vi "DateToHex.vi"(11 "DATE":timestamp[](array[timestamp])) -> (3 "数组":u16[](array[numeric]) format="%04xH")   [LabVIEW 2016, in "斯坦道总磷总氮V2.lvlib"]
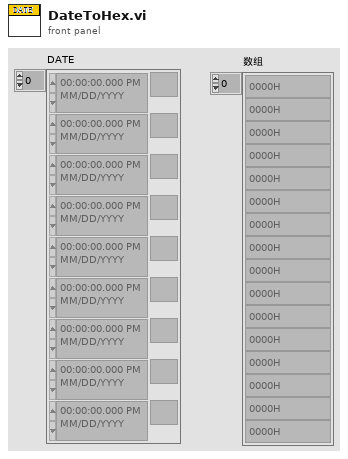
[diagram p1: front panel]
types:
  T1 = typedef "LVDateTimeRec.ctl" = cluster{"秒数的小数部分":dbl, "秒":i32, "分":i32, "时":i32, "日":i32, "月":i32, "年":i32, "天数（周）":i32, "天数（年）":i32, "DST":i32}
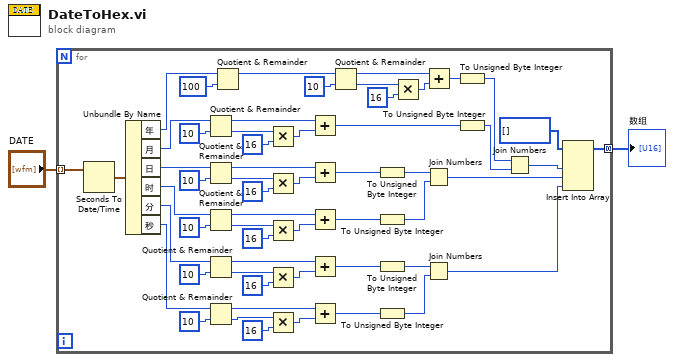
[diagram p0: block diagram]
diagram:
  n1 = for {
    tunnel: "DATE" -> [w59] mode=indexing
    tunnel: [w3] -> w1 mode=concatenating
    n2 = Seconds To Date/Time(time stamp (now)=w59) -> (date time rec=w58:T1)  [unwired: 1 in]
    n3 = Unbundle By Name(w58) -> ("年"=w26:i32, "月"=w14:i32, "日"=w13:i32, "时"=w12:i32, "分"=w11:i32, "秒"=w10:i32)
    n4 = Quotient & Remainder(x=w14, y=10) -> (x-y*floor(x/y)=w33:i32, floor(x/y)=w36:i32)
    n5 = Quotient & Remainder(x=w13, y=10) -> (x-y*floor(x/y)=w43:i32, floor(x/y)=w46:i32)
    n6 = Quotient & Remainder(x=w12, y=10) -> (x-y*floor(x/y)=w42:i32, floor(x/y)=w39:i32)
    n7 = Quotient & Remainder(x=w11, y=10) -> (x-y*floor(x/y)=w53:i32, floor(x/y)=w56:i32)
    n8 = Quotient & Remainder(x=w10, y=10) -> (x-y*floor(x/y)=w52:i32, floor(x/y)=w49:i32)
    n9 = Quotient & Remainder(x=w26, y=100) -> (x-y*floor(x/y)=w25:i32)  [unwired: 1 out]
    n10 = Multiply(x=w36, y=16) -> (x*y=w34:i32)
    n11 = Multiply(x=w46, y=16) -> (x*y=w44:i32)
    n12 = Multiply(x=w39, y=16) -> (x*y=w41:i32)
    n13 = Multiply(x=w56, y=16) -> (x*y=w54:i32)
    n14 = Multiply(x=w49, y=16) -> (x*y=w51:i32)
    n15 = Add(x=w33, y=w34) -> (x+y=w16:i32)
    n16 = Add(x=w43, y=w44) -> (x+y=w18:i32)
    n17 = Add(x=w42, y=w41) -> (x+y=w17:i32)
    n18 = Add(x=w53, y=w54) -> (x+y=w24:i32)
    n19 = Add(x=w52, y=w51) -> (x+y=w23:i32)
    n20 = Quotient & Remainder(x=w25, y=10) -> (x-y*floor(x/y)=w32:i32, floor(x/y)=w29:i32)
    n21 = To Unsigned Byte Integer(number=w18) -> (unsigned 8bit integer=w20:u8)
    n22 = To Unsigned Byte Integer(number=w17) -> (unsigned 8bit integer=w19:u8)
    n23 = To Unsigned Byte Integer(number=w24) -> (unsigned 8bit integer=w21:u8)
    n24 = To Unsigned Byte Integer(number=w23) -> (unsigned 8bit integer=w22:u8)
    n25 = Multiply(x=w29, y=16) -> (x*y=w31:i32)
    n26 = Add(x=w32, y=w31) -> (x+y=w15:i32)
    n27 = Join Numbers(hi=w20, lo=w19) -> ((hi.lo)=w5:u16)
    n28 = Join Numbers(hi=w21, lo=w22) -> ((hi.lo)=w4:u16)
    n29 = To Unsigned Byte Integer(number=w15) -> (unsigned 8bit integer=w9:u8)
    n30 = To Unsigned Byte Integer(number=w16) -> (unsigned 8bit integer=w8:u8)
    n31 = Join Numbers(hi=w9, lo=w8) -> ((hi.lo)=w7:u16)
    n32 = Insert Into Array(array=u16[] [] ("数组"), new element #1=w7, new element #2=w5, new element #3=w4) -> (w3:u16[])  [unwired: 1 in]
  }
  "数组" <- w1
